vi "receiveUdp.vi"() -> ()   [LabVIEW 2021]
uses:
  Jump_Globals.vi
  senzorji.vi
  Jumps_Globals.vi
  Stevci_Globals.vi
  filePath.vi
  belezenje.vi
  <vilib>/express/express arith-compare/Formula/XNode/ExpressFormulaBlockNode.xnode
panel:
  out "Whole packet  3":string
  out "Whole packet  2":string
  out "Whole packet  1":string
  out "Whole packet 6  2":string
  out "Whole packet 5  2":string
  out "Whole packet  4":string
  out "Numeric":dbl
  out "appended path":path
  out "Jump ID 6":string
  out "Jump time  6":string
  out "Flight time 6":string
  out "Battery  6":string
  out "Sensor ID   6":string
  out "Packet Time 6":string
  out "appended path 6":path
  out "Jump ID 5":string
  out "Jump time  5":string
  out "Flight time 5":string
  out "Battery  5":string
  out "Sensor ID   5":string
  out "Packet Time 5":string
  out "appended path 5":path
  out "Jump ID 4":string
  out "Jump time  4":string
  out "Flight time 4":string
  out "Battery  4":string
  out "Sensor ID   4":string
  out "Packet Time 4":string
  out "appended path 4":path
  out "Jump ID 3":string
  out "Jump time  3":string
  out "Flight time 3":string
  out "Battery  3":string
  out "Sensor ID   3":string
  out "Packet Time 3":string
  out "Jump ID 2":string
  out "Jump time  2":string
  out "Flight time 2":string
  out "Battery  2":string
  out "Sensor ID   2":string
  out "Packet Time  2":string
  out "appended path 2":path
  out "Packet Time":string
  out "Sensor ID":string
  out "Whole packet":string
  out "Battery":string
  out "Flight time":string
  out "Jump time":string
  out "Jump ID":string
  in  "Stop":bool
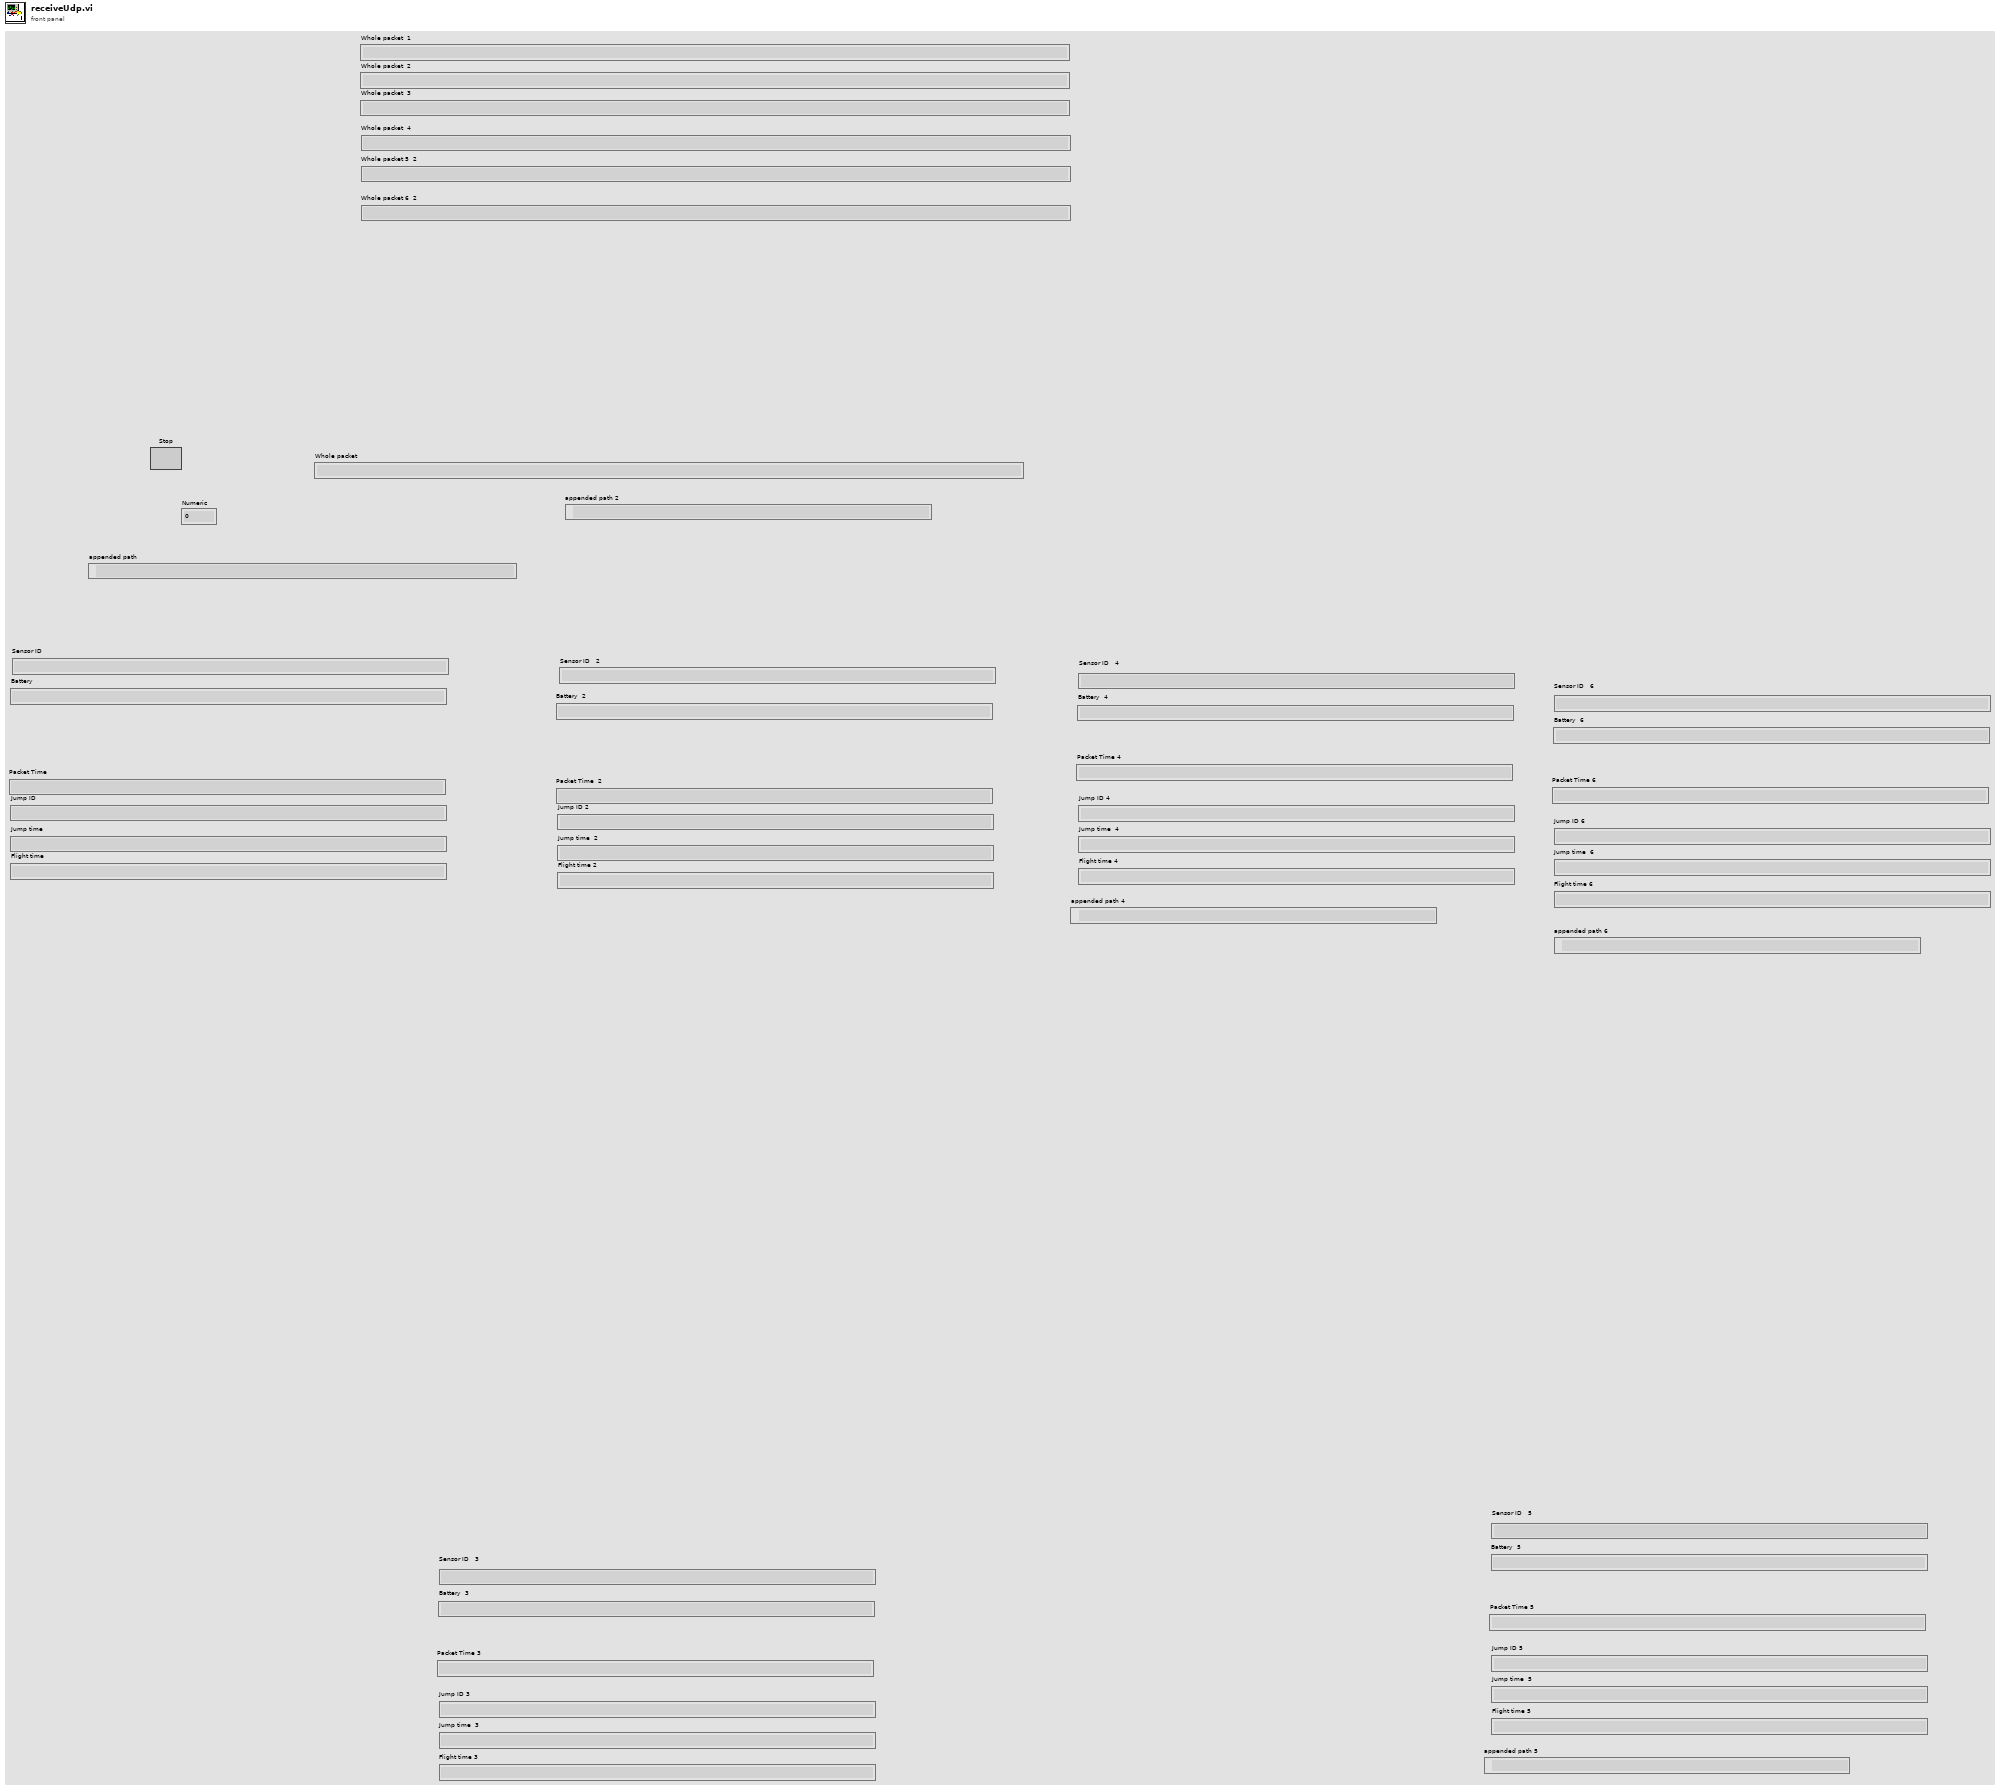
[diagram p1: front panel]
types:
  T1 = enum16{"open", "open or create", "create or replace", "create", "open (read-only)"}
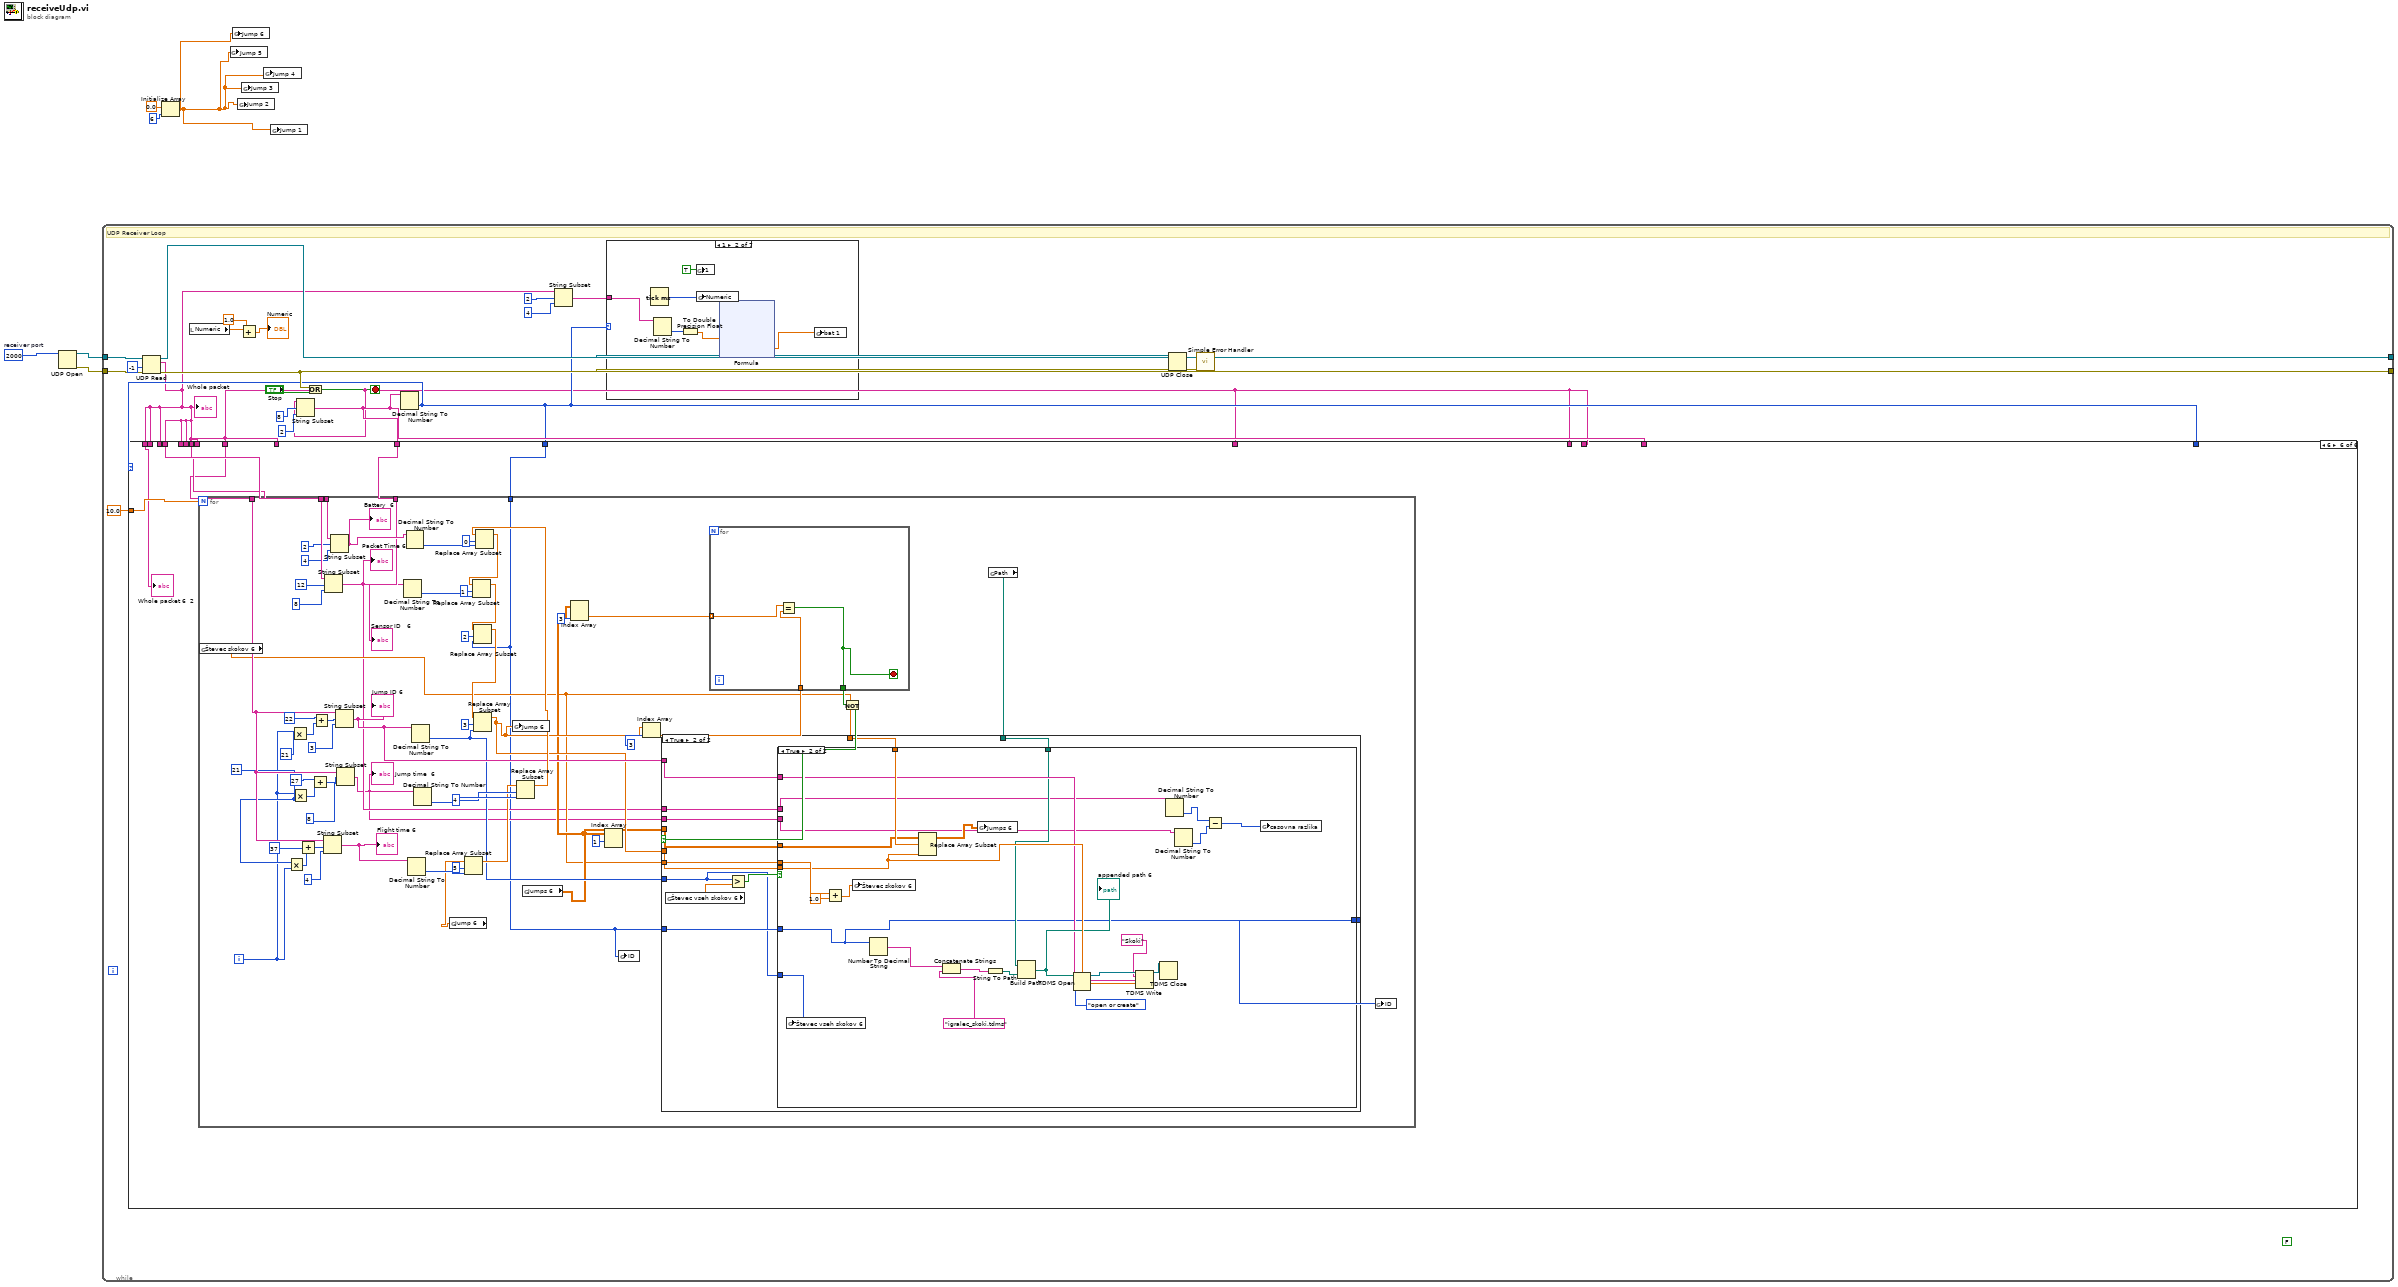
[diagram p0: block diagram]
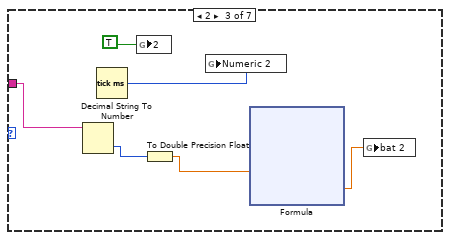
[diagram p3: hidden frame]
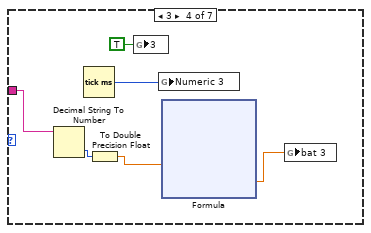
[diagram p4: hidden frame]
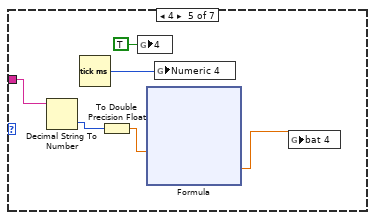
[diagram p5: hidden frame]
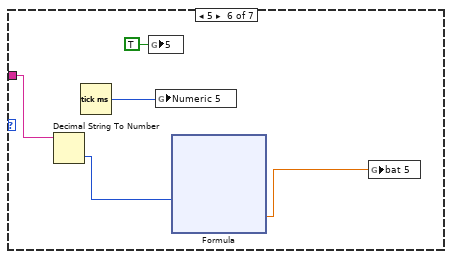
[diagram p6: hidden frame]
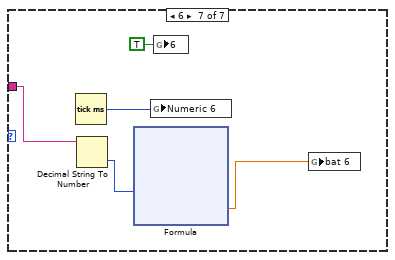
[diagram p7: hidden frame]
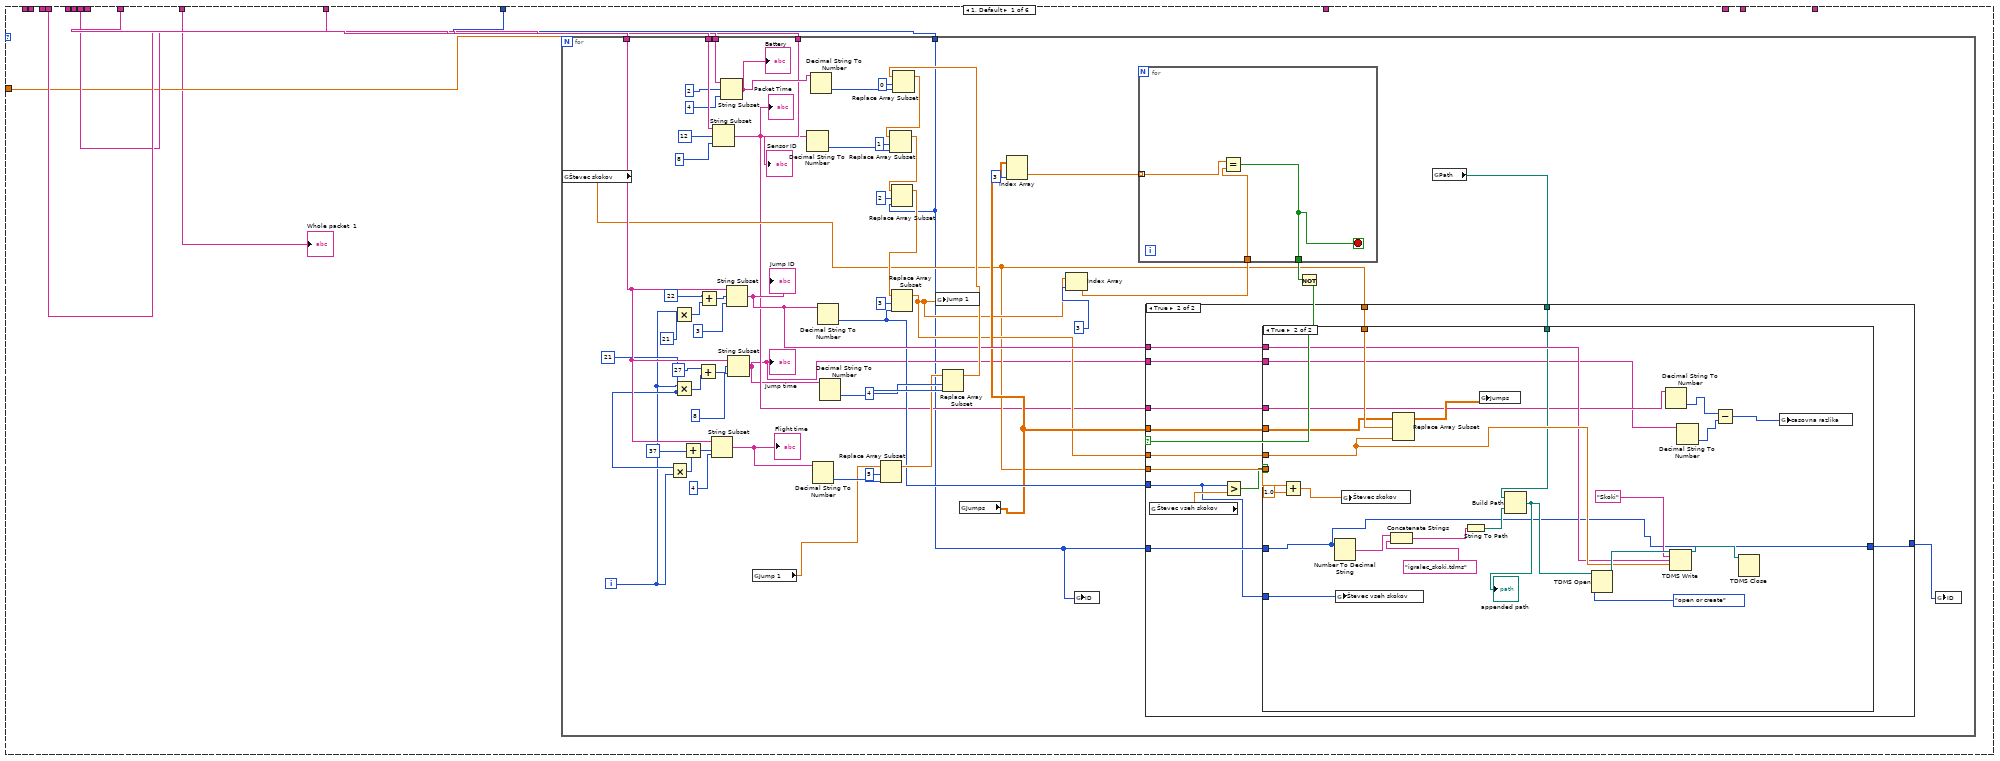
[diagram p8: hidden frame]
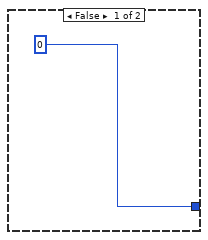
[diagram p9: hidden frame]
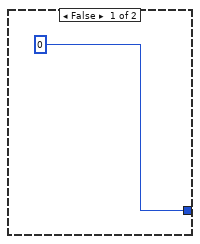
[diagram p10: hidden frame]
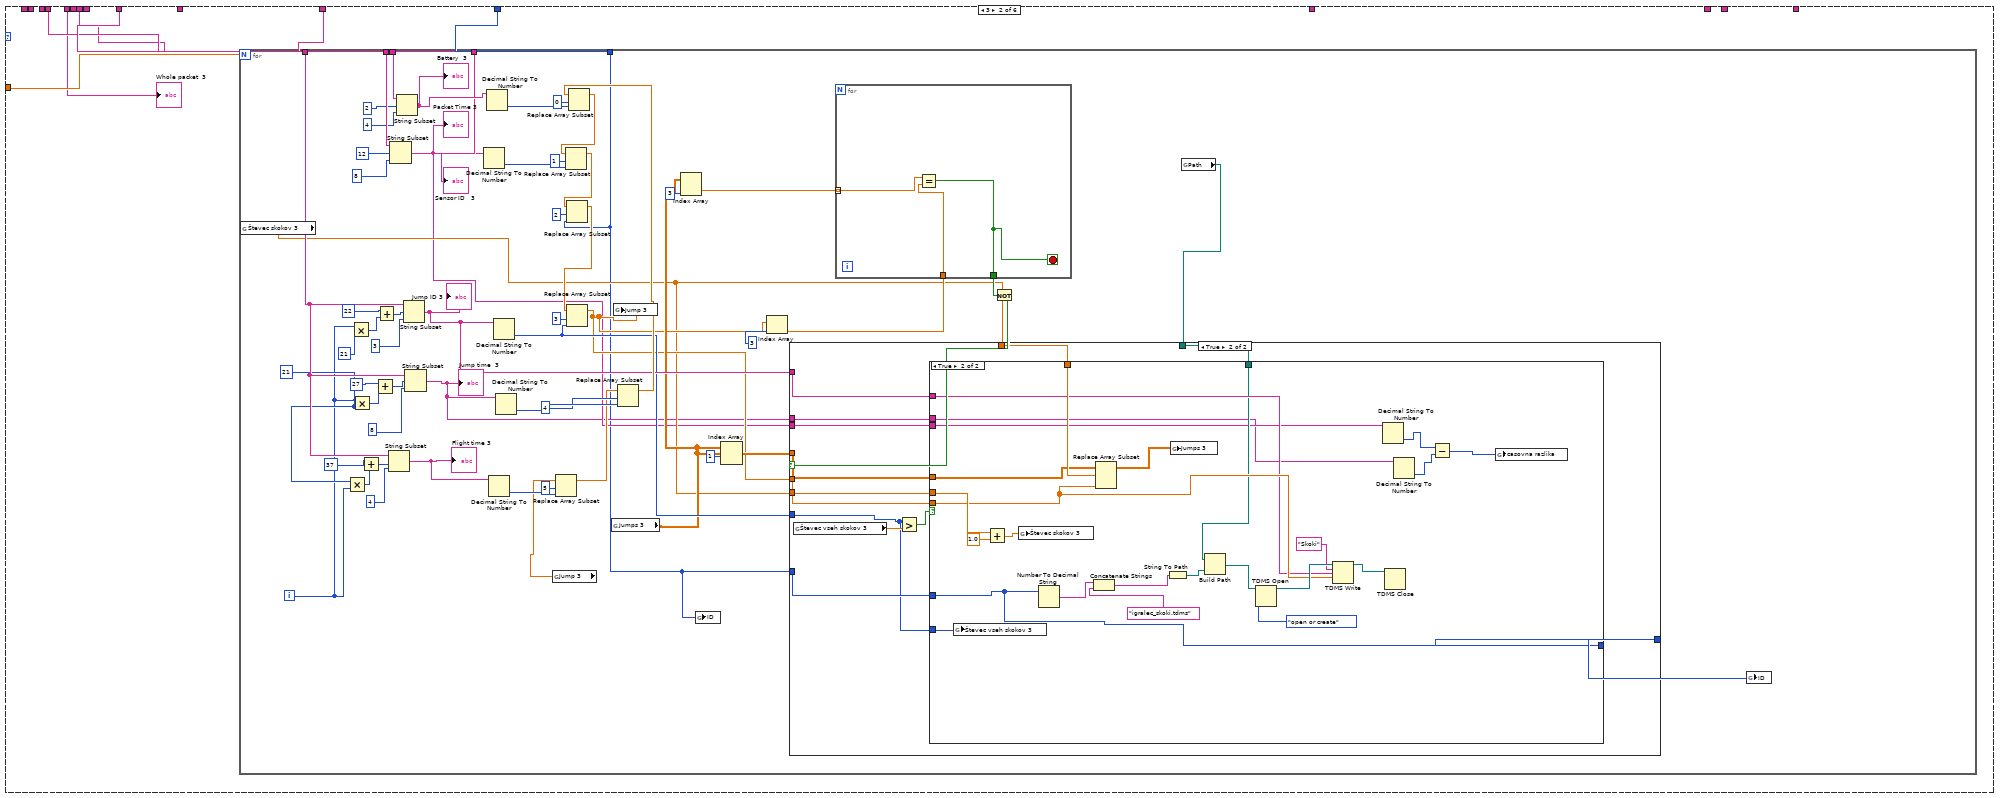
[diagram p11: hidden frame]
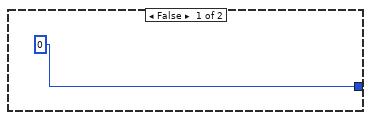
[diagram p12: hidden frame]
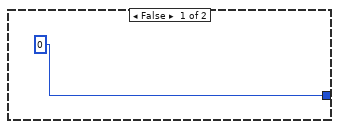
[diagram p13: hidden frame]
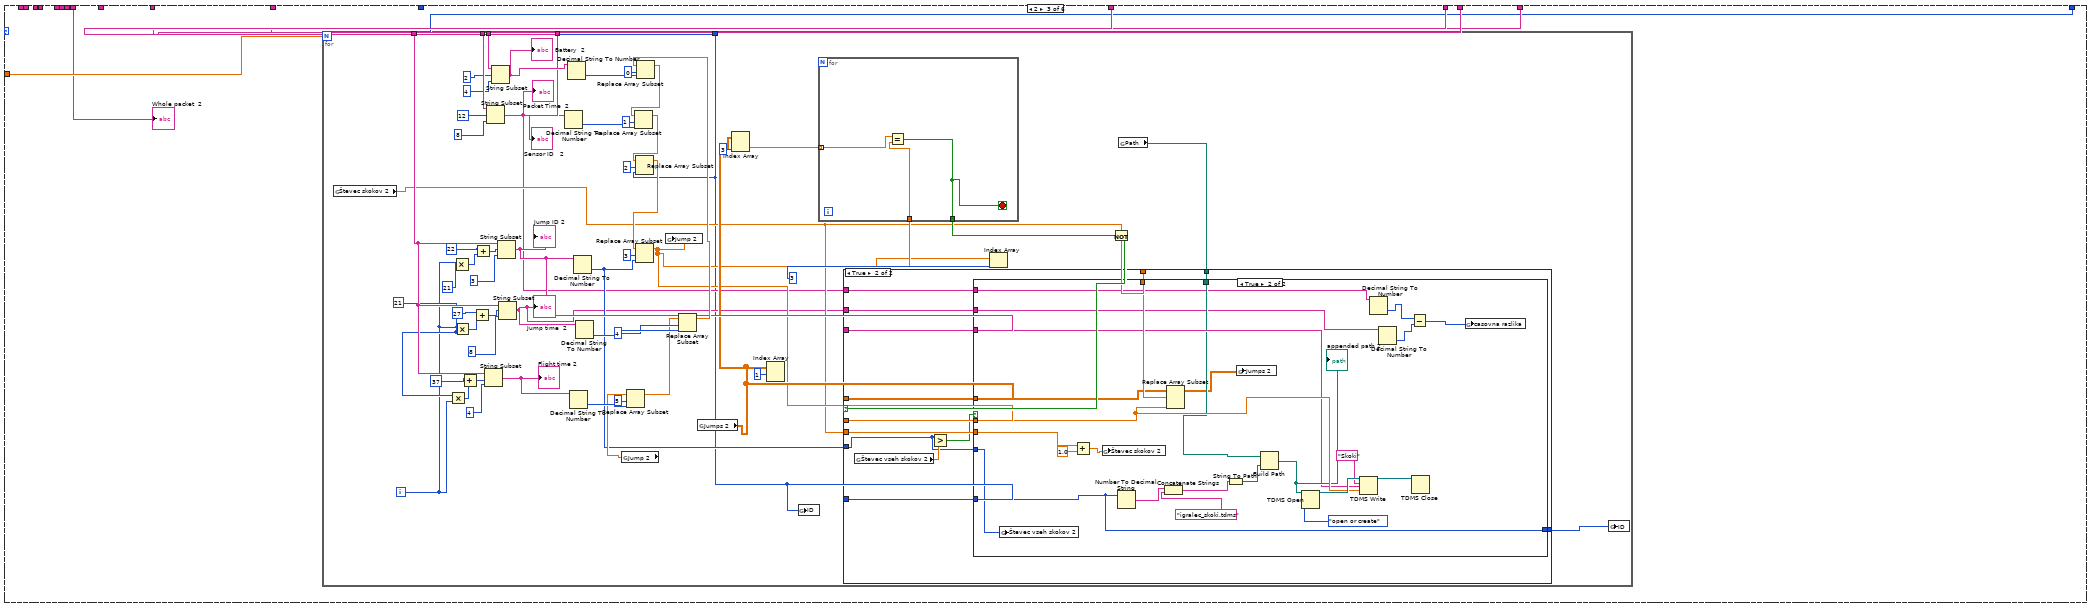
[diagram p14: hidden frame]
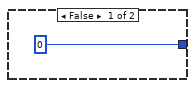
[diagram p15: hidden frame]
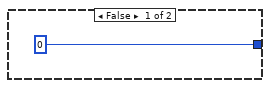
[diagram p16: hidden frame]
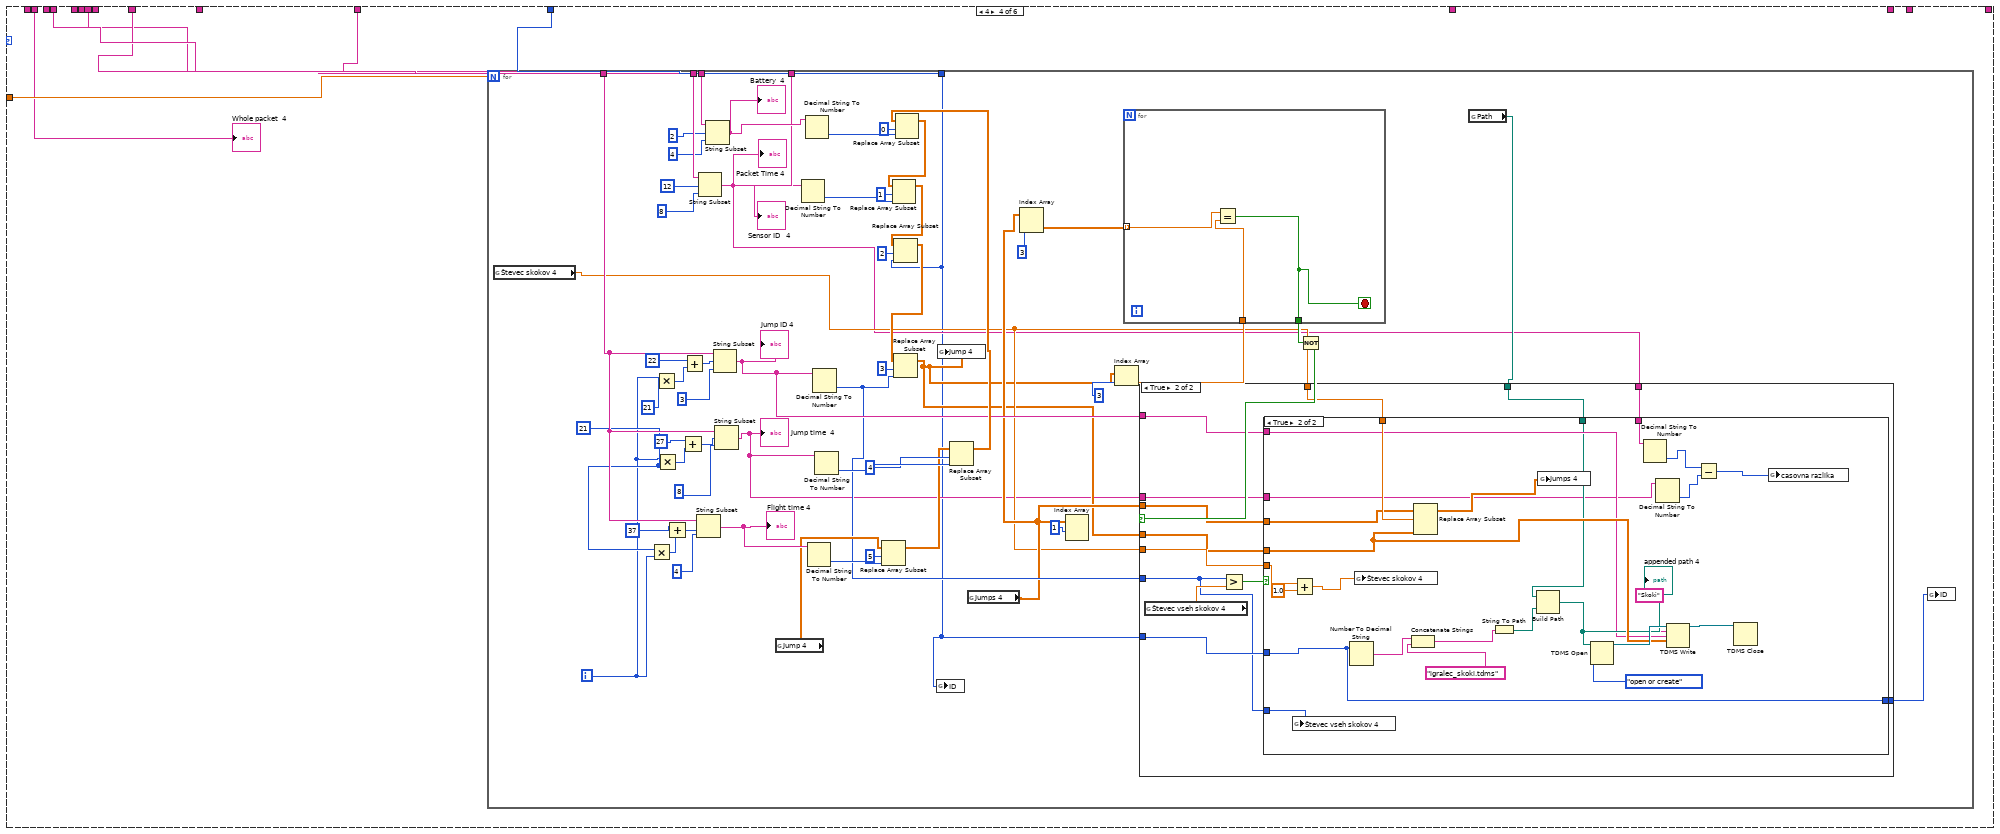
[diagram p17: hidden frame]
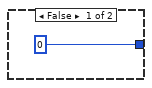
[diagram p18: hidden frame]
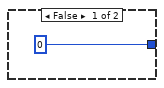
[diagram p19: hidden frame]
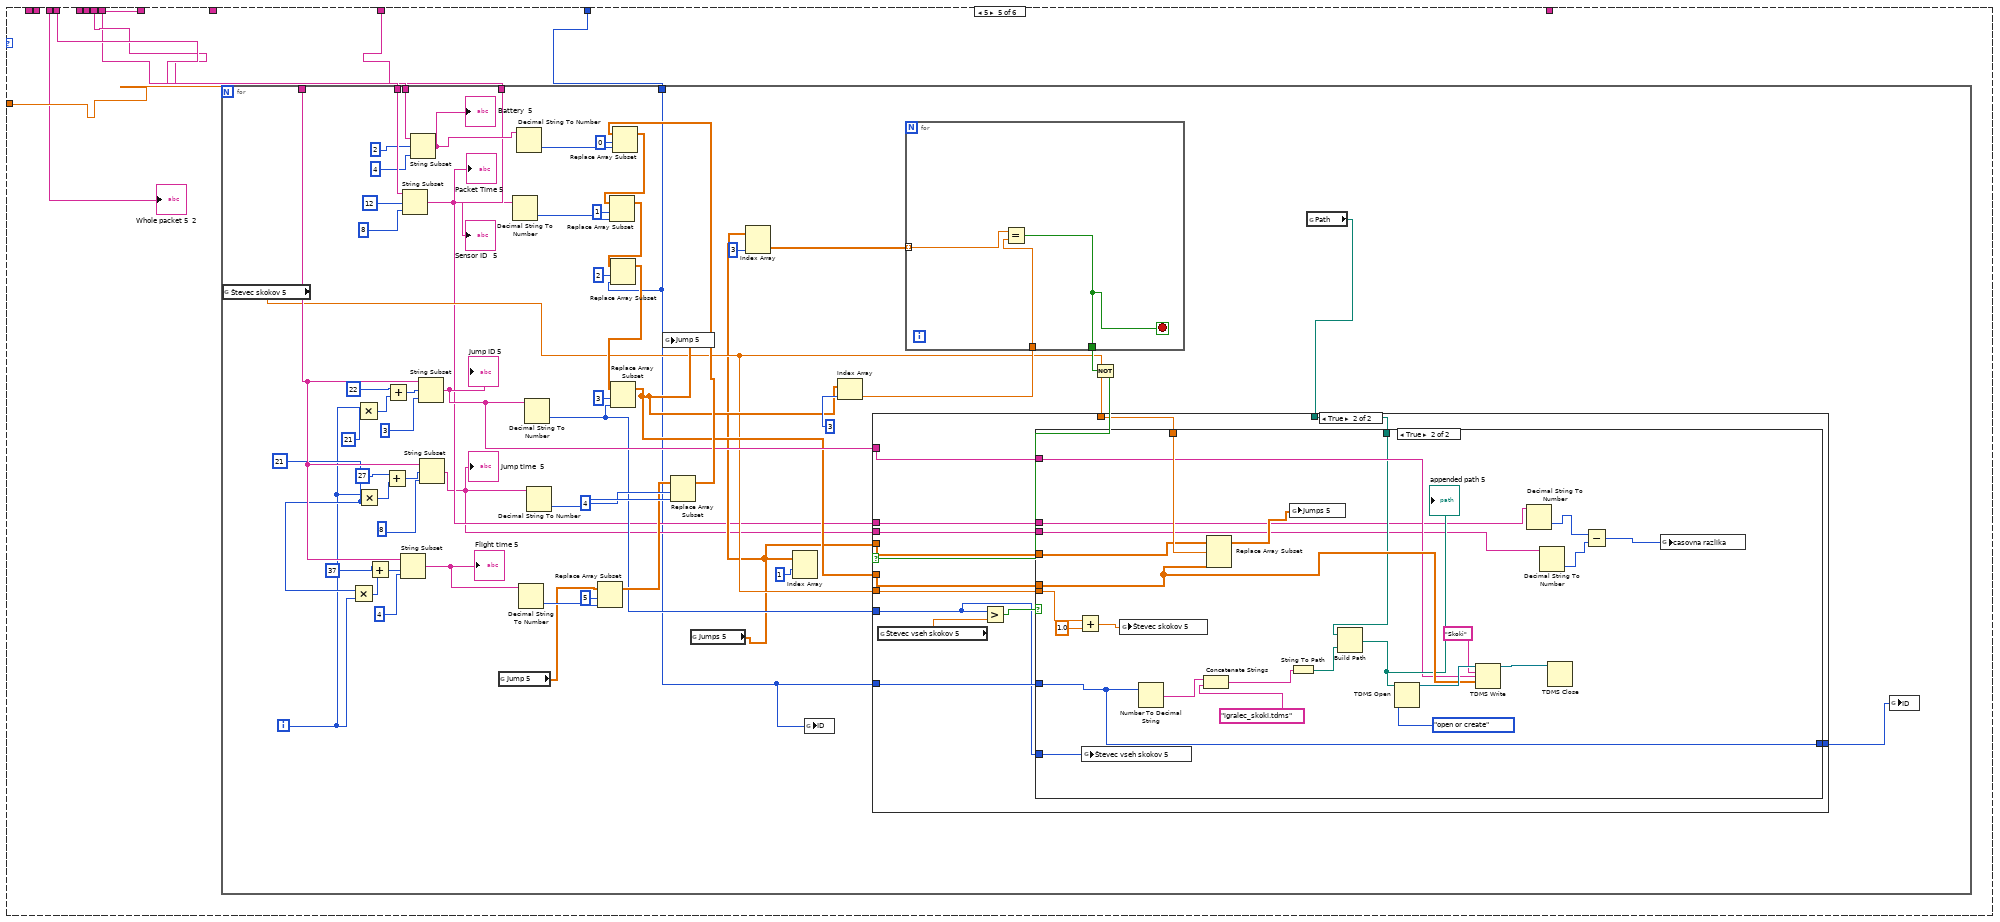
[diagram p20: hidden frame]
diagram:
  w2 = u16 2000  # receiver port
  n1 = UDP Open(11:w2) -> (port=w3:refnum<k16>, 0:w4:errorcluster)  [unwired: 4 in, 1 out]
  n2 = while {
    tunnel: w3 -> [w28]
    tunnel: [w24] -> w7
    tunnel: w4 -> [w25]
    tunnel: [w23] -> w5
    stop <- w26 stop-if-true
    (unwired) FALSE
    # "UDP Receiver Loop"
    n3 = UDP Read(connection ID=w28, timeout ms (25000)=-1, 8:w25) -> (data out=w10:string, error out=w23:errorcluster, 3:w24:refnum<k16>)  [unwired: 3 out]
    "Whole packet" <- w10
    n4 = local read "Numeric"() -> (w13:dbl)
    n5 = Add(x=w13, y=1.0) -> (x+y=→"Numeric":dbl)
    n6 = String Subset(string=w10, offset (0)=8, length (rest)=2) -> (substring=w20:string)
    n7 = Or(x=w23, y="Stop") -> (x .or. y?=w26:bool)
    n8 = Decimal String To Number(string=w20) -> (number=w17:i32)  [unwired: 2 in, 1 out]
    n9 = case shown="6" w17 {
      tunnel: w10 -> [w117 w223 _ w438 w546 w653]
      tunnel: w10 -> [w116 w222 _ w436 w548 w656]
      tunnel: w10 -> [w115 w221 _ w439 w547 w654]
      tunnel: w20 -> [w114 w220 _ w437 w544 w652]
      tunnel: w17 -> [w113 w224 _ w440 w545 w655]
      tunnel: w10 -> [_ _ w332 _ _ _]
      tunnel: w10 -> [_ _ w331 _ _ _]
      tunnel: w10 -> [_ _ w330 _ _ _]
      tunnel: w20 -> [_ _ w329 _ _ _]
      tunnel: w17 -> [_ _ w328 _ _ _]
      tunnel: 10.0 ("Numeric") -> [w112 w219 w327 w435 w543 w651]
      tunnel: w10 -> [w111 _ _ _ _ _]
      tunnel: w10 -> [_ _ _ _ _ _]
      tunnel: w10 -> [_ w218 _ _ _ _]
      tunnel: w10 -> [_ _ w326 _ _ _]
      tunnel: w10 -> [_ _ _ w434 _ _]
      tunnel: w10 -> [_ _ _ _ w542 _]
      tunnel: w10 -> [_ _ _ _ _ w650]
      frame 1, Default {
        n10 = for {
          N: w112 -> [_]
          tunnel: w117 -> [w171]
          tunnel: w116 -> [w148]
          tunnel: w115 -> [w145]
          tunnel: w114 -> [w128]
          tunnel: w113 -> [w118]
          i -> [w131]
          w163 = 21
          n11 = global read "Stevci_Globals.vi" "Števec skokov"() -> (w122:dbl)
          n12 = Multiply(x=w163, y=w131) -> (x*y=w166:i32)
          n13 = Multiply(x=21, y=w131) -> (x*y=w168:i32)
          n14 = Multiply(x=w131, y=w163) -> (x*y=w170:i32)
          n15 = Add(x=37, y=w166) -> (x+y=w165:i32)
          n16 = Add(x=27, y=w170) -> (x+y=w161:i32)
          n17 = Add(x=22, y=w168) -> (x+y=w160:i32)
          n18 = String Subset(string=w171, offset (0)=w165, length (rest)=4) -> (substring=w159:string)
          "Flight time" <- w159
          n19 = String Subset(string=w148, offset (0)=12, length (rest)=8) -> (substring=w120:string)
          "Packet Time" <- w120
          n20 = String Subset(string=w145, offset (0)=2, length (rest)=4) -> (substring=w137:string)
          "Battery" <- w137
          n21 = String Subset(string=w171, offset (0)=w160, length (rest)=3) -> (substring=w129:string)
          "Jump ID" <- w129
          n22 = String Subset(string=w171, offset (0)=w161, length (rest)=8) -> (substring=w119:string)
          "Jump time" <- w119
          n23 = global read "Jump_Globals.vi" "Jump 1"() -> (w124:dbl[])
          n24 = Decimal String To Number(string=w120) -> (number=w152:i32)  [unwired: 2 in, 1 out]
          n25 = Decimal String To Number(string=w137) -> (number=w151:i32)  [unwired: 2 in, 1 out]
          n26 = Decimal String To Number(string=w159) -> (number=w157:i32)  [unwired: 2 in, 1 out]
          n27 = Decimal String To Number(string=w129) -> (number=w127:i32)  [unwired: 2 in, 1 out]
          n28 = Decimal String To Number(string=w119) -> (number=w158:i32)  [unwired: 2 in, 1 out]
          n29 = Replace Array Subset(array=w124, new element=w157, index=5) -> (w153:dbl[])
          n30 = Replace Array Subset(array=w153, new element=w158, index=4) -> (w144:dbl[])
          n31 = Replace Array Subset(array=w144, new element=w151, index=0) -> (w143:dbl[])
          n32 = Replace Array Subset(array=w143, new element=w152, index=1) -> (w142:dbl[])
          n33 = Replace Array Subset(array=w142, new element=w118, index=2) -> (w141:dbl[])
          n34 = Replace Array Subset(array=w141, new element=w127, index=3) -> (w123:dbl[])
          n35 = global write "Jump_Globals.vi" "Jump 1"(w123) -> ()
          n36 = global read "Jumps_Globals.vi" "Jumps"() -> (w125:dbl[][])
          n37 = Index Array(array=w125, index (col)=3 ("disabled index (col)")) -> (element=w135:dbl[])  [unwired: 1 in]
          n38 = Index Array(array=w123, index=3) -> (element=w133:dbl)
          n39 = global write "belezenje.vi" "ID"(w118) -> ()
          n40 = for {
            tunnel: w135 -> [w217] mode=indexing
            tunnel: w133 -> [w216]
            tunnel: [w215] -> w132
            stop <- w215 stop-if-true
            n41 = Equal?(x=w217, y=w216) -> (x = y?=w215:bool)
          }
          n42 = Not(x=w132) -> (.not. x?=w130:bool)
          n43 = global read "filePath.vi" "Path"() -> (w121:path)
          n44 = case shown="True" w130 {
            tunnel: w125 -> [_ w186]
            tunnel: w123 -> [_ w185]
            tunnel: w122 -> [_ w188]
            tunnel: w122 -> [_ w187]
            tunnel: w129 -> [_ w184]
            tunnel: w118 -> [_ w183]
            tunnel: w121 -> [_ w182]
            tunnel: w127 -> [_ w179]
            tunnel: [0 w178] -> w126
            tunnel: w120 -> [_ w177]
            tunnel: w119 -> [_ w176]
            frame False {
            }
            frame True {
              n45 = global read "Stevci_Globals.vi" "Števec vseh skokov"() -> (w181:dbl)
              n46 = Greater?(x=w179, y=w181) -> (0:w180:bool)
              n47 = case shown="True" w180 {
                tunnel: w188 -> [_ w214]
                tunnel: w187 -> [_ w213]
                tunnel: w186 -> [_ w208]
                tunnel: w185 -> [_ w207]
                tunnel: w184 -> [_ w204]
                tunnel: w183 -> [_ w195]
                tunnel: w182 -> [_ w199]
                tunnel: w179 -> [_ w196]
                tunnel: [0 w195] -> w178
                tunnel: w177 -> [_ w191]
                tunnel: w176 -> [_ w190]
                frame False {
                }
                frame True {
                  n48 = Add(x=w213, y=1.0) -> (x+y=w197:dbl)
                  n49 = Number To Decimal String(number=w195) -> (decimal integer string=w203:string)  [unwired: 1 in]
                  n50 = global write "Stevci_Globals.vi" "Števec vseh skokov"(w196) -> ()
                  n51 = global write "Stevci_Globals.vi" "Števec skokov"(w197) -> ()
                  n52 = Concatenate Strings(w203, "igralec_skoki.tdms") -> (w201:string)
                  n53 = Replace Array Subset(array=w208, new element=w207, index (row)=w214) -> (w198:dbl[][])  [unwired: 1 in]
                  n54 = String To Path(string=w201) -> (path=w200:path)
                  n55 = global write "Jumps_Globals.vi" "Jumps"(w198) -> ()
                  n56 = Build Path(base path=w199, name or relative path=w200) -> (appended path=w206:path)
                  "appended path" <- w206
                  n57 = TDMS Open(10:T1."open or create" ("operation (0:open)"), 11:w206) -> (3:w211:refnum<k34>)  [unwired: 5 in, 1 out]
                  n58 = Decimal String To Number(string=w191) -> (number=w193:i32)  [unwired: 2 in, 1 out]
                  n59 = TDMS Write(0:w211, 5:"Skoki" ("group name in (Untitled)"), 7:w204, 9:w207) -> (4:w210:refnum<k34>)  [unwired: 2 in, 3 out]
                  n60 = Decimal String To Number(string=w190) -> (number=w192:i32)  [unwired: 2 in, 1 out]
                  n61 = Subtract(x=w193, y=w192) -> (x-y=w194:i32)
                  n62 = TDMS Close(11:w210) -> ()  [unwired: 1 in, 2 out]
                  n63 = global write "Stevci_Globals.vi" "casovna razlika"(w194) -> ()
                }
              }
            }
          }
          n64 = global write "belezenje.vi" "ID"(w126) -> ()
          "Sensor ID" <- w128
        }
        "Whole packet  1" <- w111
      }
      frame 3 {
        n65 = for {
          N: w219 -> [_]
          tunnel: w223 -> [w279]
          tunnel: w222 -> [w255]
          tunnel: w221 -> [w252]
          tunnel: w220 -> [w235]
          tunnel: w224 -> [w225]
          i -> [w238]
          w271 = 21
          n66 = global read "Stevci_Globals.vi" "Števec skokov 3"() -> (w229:dbl)
          n67 = Multiply(x=w271, y=w238) -> (x*y=w274:i32)
          n68 = Multiply(x=21, y=w238) -> (x*y=w276:i32)
          n69 = Multiply(x=w238, y=w271) -> (x*y=w278:i32)
          n70 = Add(x=37, y=w274) -> (x+y=w273:i32)
          n71 = Add(x=27, y=w278) -> (x+y=w269:i32)
          n72 = Add(x=22, y=w276) -> (x+y=w268:i32)
          n73 = String Subset(string=w279, offset (0)=w273, length (rest)=4) -> (substring=w267:string)
          "Flight time 3" <- w267
          n74 = String Subset(string=w255, offset (0)=12, length (rest)=8) -> (substring=w227:string)
          "Packet Time 3" <- w227
          n75 = String Subset(string=w252, offset (0)=2, length (rest)=4) -> (substring=w244:string)
          "Battery  3" <- w244
          n76 = String Subset(string=w279, offset (0)=w268, length (rest)=3) -> (substring=w236:string)
          "Jump ID 3" <- w236
          n77 = String Subset(string=w279, offset (0)=w269, length (rest)=8) -> (substring=w226:string)
          "Jump time  3" <- w226
          n78 = Decimal String To Number(string=w227) -> (number=w259:i32)  [unwired: 2 in, 1 out]
          n79 = Decimal String To Number(string=w244) -> (number=w258:i32)  [unwired: 2 in, 1 out]
          n80 = Decimal String To Number(string=w267) -> (number=w265:i32)  [unwired: 2 in, 1 out]
          n81 = Decimal String To Number(string=w236) -> (number=w233:i32)  [unwired: 2 in, 1 out]
          n82 = Decimal String To Number(string=w226) -> (number=w266:i32)  [unwired: 2 in, 1 out]
          n83 = global read "Jump_Globals.vi" "Jump 3"() -> (w234:dbl[])
          n84 = Replace Array Subset(array=w234, new element=w265, index=5) -> (w261:dbl[])
          n85 = global read "Jumps_Globals.vi" "Jumps 3"() -> (w231:dbl[][])
          n86 = Replace Array Subset(array=w261, new element=w266, index=4) -> (w251:dbl[])
          n87 = Replace Array Subset(array=w251, new element=w258, index=0) -> (w250:dbl[])
          n88 = Replace Array Subset(array=w250, new element=w259, index=1) -> (w249:dbl[])
          n89 = Replace Array Subset(array=w249, new element=w225, index=2) -> (w248:dbl[])
          n90 = Replace Array Subset(array=w248, new element=w233, index=3) -> (w230:dbl[])
          n91 = global write "Jump_Globals.vi" "Jump 3"(w230) -> ()
          n92 = Index Array(array=w231, index (col)=3 ("disabled index (col)")) -> (element=w242:dbl[])  [unwired: 1 in]
          n93 = global write "belezenje.vi" "ID"(w225) -> ()
          n94 = Index Array(array=w231, index (row)=1) -> ()  [unwired: 1 in, 1 out]
          n95 = Index Array(array=w230, index=3) -> (element=w240:dbl)
          n96 = for {
            tunnel: w242 -> [w325] mode=indexing
            tunnel: w240 -> [w324]
            tunnel: [w323] -> w239
            stop <- w323 stop-if-true
            n97 = Equal?(x=w325, y=w324) -> (x = y?=w323:bool)
          }
          n98 = Not(x=w239) -> (.not. x?=w237:bool)
          n99 = global read "filePath.vi" "Path"() -> (w228:path)
          n100 = case shown="True" w237 {
            tunnel: w231 -> [_ w294]
            tunnel: w230 -> [_ w293]
            tunnel: w229 -> [_ w296]
            tunnel: w229 -> [_ w295]
            tunnel: w236 -> [_ w292]
            tunnel: w225 -> [_ w291]
            tunnel: w228 -> [_ w290]
            tunnel: w233 -> [_ w287]
            tunnel: [0 w286] -> w232
            tunnel: w227 -> [_ w285]
            tunnel: w226 -> [_ w284]
            frame False {
            }
            frame True {
              n101 = global read "Stevci_Globals.vi" "Števec vseh skokov 3"() -> (w289:dbl)
              n102 = Greater?(x=w287, y=w289) -> (0:w288:bool)
              n103 = case shown="True" w288 {
                tunnel: w296 -> [_ w322]
                tunnel: w295 -> [_ w321]
                tunnel: w294 -> [_ w316]
                tunnel: w293 -> [_ w315]
                tunnel: w292 -> [_ w312]
                tunnel: w291 -> [_ w303]
                tunnel: w290 -> [_ w307]
                tunnel: w287 -> [_ w305]
                tunnel: [0 w303] -> w286
                tunnel: w285 -> [_ w299]
                tunnel: w284 -> [_ w298]
                frame False {
                }
                frame True {
                  n104 = global write "Stevci_Globals.vi" "Števec vseh skokov 3"(w305) -> ()
                  n105 = Add(x=w321, y=1.0) -> (x+y=w304:dbl)
                  n106 = global write "Stevci_Globals.vi" "Števec skokov 3"(w304) -> ()
                  n107 = Number To Decimal String(number=w303) -> (decimal integer string=w311:string)  [unwired: 1 in]
                  n108 = Concatenate Strings(w311, "igralec_skoki.tdms") -> (w309:string)
                  n109 = Replace Array Subset(array=w316, new element=w315, index (row)=w322) -> (w306:dbl[][])  [unwired: 1 in]
                  n110 = String To Path(string=w309) -> (path=w308:path)
                  n111 = global write "Jumps_Globals.vi" "Jumps 3"(w306) -> ()
                  n112 = Build Path(base path=w307, name or relative path=w308) -> (appended path=w314:path)
                  n113 = TDMS Open(10:T1."open or create" ("operation (0:open)"), 11:w314) -> (3:w319:refnum<k34>)  [unwired: 5 in, 1 out]
                  n114 = TDMS Write(0:w319, 5:"Skoki" ("group name in (Untitled)"), 7:w312, 9:w315) -> (4:w318:refnum<k34>)  [unwired: 2 in, 3 out]
                  n115 = Decimal String To Number(string=w299) -> (number=w301:i32)  [unwired: 2 in, 1 out]
                  n116 = TDMS Close(11:w318) -> ()  [unwired: 1 in, 2 out]
                  n117 = Decimal String To Number(string=w298) -> (number=w300:i32)  [unwired: 2 in, 1 out]
                  n118 = Subtract(x=w301, y=w300) -> (x-y=w302:i32)
                  n119 = global write "Stevci_Globals.vi" "casovna razlika"(w302) -> ()
                }
              }
            }
          }
          n120 = global write "belezenje.vi" "ID"(w232) -> ()
          "Sensor ID   3" <- w235
        }
        "Whole packet  3" <- w218
      }
      frame 2 {
        n121 = for {
          N: w327 -> [_]
          tunnel: w332 -> [w387]
          tunnel: w331 -> [w363]
          tunnel: w330 -> [w360]
          tunnel: w329 -> [w343]
          tunnel: w328 -> [w333]
          i -> [w346]
          w379 = 21
          n122 = global read "Stevci_Globals.vi" "Števec skokov 2"() -> (w337:dbl)
          n123 = Multiply(x=w379, y=w346) -> (x*y=w382:i32)
          n124 = Multiply(x=21, y=w346) -> (x*y=w384:i32)
          n125 = Multiply(x=w346, y=w379) -> (x*y=w386:i32)
          n126 = Add(x=37, y=w382) -> (x+y=w381:i32)
          n127 = Add(x=27, y=w386) -> (x+y=w377:i32)
          n128 = Add(x=22, y=w384) -> (x+y=w376:i32)
          n129 = String Subset(string=w387, offset (0)=w381, length (rest)=4) -> (substring=w375:string)
          "Flight time 2" <- w375
          n130 = String Subset(string=w363, offset (0)=12, length (rest)=8) -> (substring=w335:string)
          "Packet Time  2" <- w335
          n131 = String Subset(string=w360, offset (0)=2, length (rest)=4) -> (substring=w352:string)
          "Battery  2" <- w352
          n132 = String Subset(string=w387, offset (0)=w376, length (rest)=3) -> (substring=w344:string)
          "Jump ID 2" <- w344
          n133 = String Subset(string=w387, offset (0)=w377, length (rest)=8) -> (substring=w334:string)
          "Jump time  2" <- w334
          n134 = Decimal String To Number(string=w335) -> (number=w367:i32)  [unwired: 2 in, 1 out]
          n135 = Decimal String To Number(string=w352) -> (number=w366:i32)  [unwired: 2 in, 1 out]
          n136 = Decimal String To Number(string=w375) -> (number=w373:i32)  [unwired: 2 in, 1 out]
          n137 = Decimal String To Number(string=w344) -> (number=w341:i32)  [unwired: 2 in, 1 out]
          n138 = Decimal String To Number(string=w334) -> (number=w374:i32)  [unwired: 2 in, 1 out]
          n139 = global read "Jump_Globals.vi" "Jump 2"() -> (w342:dbl[])
          n140 = Replace Array Subset(array=w342, new element=w373, index=5) -> (w369:dbl[])
          n141 = Replace Array Subset(array=w369, new element=w374, index=4) -> (w359:dbl[])
          n142 = Replace Array Subset(array=w359, new element=w366, index=0) -> (w358:dbl[])
          n143 = Replace Array Subset(array=w358, new element=w367, index=1) -> (w357:dbl[])
          n144 = Replace Array Subset(array=w357, new element=w333, index=2) -> (w356:dbl[])
          n145 = Replace Array Subset(array=w356, new element=w341, index=3) -> (w338:dbl[])
          n146 = global write "Jump_Globals.vi" "Jump 2"(w338) -> ()
          n147 = global read "Jumps_Globals.vi" "Jumps 2"() -> (w339:dbl[][])
          n148 = Index Array(array=w339, index (col)=3 ("disabled index (col)")) -> (element=w350:dbl[])  [unwired: 1 in]
          n149 = Index Array(array=w339, index (row)=1) -> ()  [unwired: 1 in, 1 out]
          n150 = global write "belezenje.vi" "ID"(w333) -> ()
          n151 = Index Array(array=w338, index=3) -> (element=w348:dbl)
          n152 = for {
            tunnel: w350 -> [w433] mode=indexing
            tunnel: w348 -> [w432]
            tunnel: [w431] -> w347
            stop <- w431 stop-if-true
            n153 = Equal?(x=w433, y=w432) -> (x = y?=w431:bool)
          }
          n154 = Not(x=w347) -> (.not. x?=w345:bool)
          n155 = global read "filePath.vi" "Path"() -> (w336:path)
          n156 = case shown="True" w345 {
            tunnel: w339 -> [_ w402]
            tunnel: w338 -> [_ w401]
            tunnel: w337 -> [_ w404]
            tunnel: w337 -> [_ w403]
            tunnel: w344 -> [_ w400]
            tunnel: w333 -> [_ w399]
            tunnel: w336 -> [_ w398]
            tunnel: w341 -> [_ w395]
            tunnel: [0 w394] -> w340
            tunnel: w335 -> [_ w393]
            tunnel: w334 -> [_ w392]
            frame False {
            }
            frame True {
              n157 = global read "Stevci_Globals.vi" "Števec vseh skokov 2"() -> (w397:dbl)
              n158 = Greater?(x=w395, y=w397) -> (0:w396:bool)
              n159 = case shown="True" w396 {
                tunnel: w404 -> [_ w430]
                tunnel: w403 -> [_ w429]
                tunnel: w402 -> [_ w424]
                tunnel: w401 -> [_ w423]
                tunnel: w400 -> [_ w420]
                tunnel: w399 -> [_ w411]
                tunnel: w398 -> [_ w415]
                tunnel: w395 -> [_ w413]
                tunnel: [0 w411] -> w394
                tunnel: w393 -> [_ w407]
                tunnel: w392 -> [_ w406]
                frame False {
                }
                frame True {
                  n160 = global write "Stevci_Globals.vi" "Števec vseh skokov 2"(w413) -> ()
                  n161 = Add(x=w429, y=1.0) -> (x+y=w412:dbl)
                  n162 = global write "Stevci_Globals.vi" "Števec skokov 2"(w412) -> ()
                  n163 = Number To Decimal String(number=w411) -> (decimal integer string=w419:string)  [unwired: 1 in]
                  n164 = Concatenate Strings(w419, "igralec_skoki.tdms") -> (w417:string)
                  n165 = Replace Array Subset(array=w424, new element=w423, index (row)=w430) -> (w414:dbl[][])  [unwired: 1 in]
                  n166 = String To Path(string=w417) -> (path=w416:path)
                  n167 = global write "Jumps_Globals.vi" "Jumps 2"(w414) -> ()
                  n168 = Build Path(base path=w415, name or relative path=w416) -> (appended path=w422:path)
                  "appended path 2" <- w422
                  n169 = TDMS Open(10:T1."open or create" ("operation (0:open)"), 11:w422) -> (3:w427:refnum<k34>)  [unwired: 5 in, 1 out]
                  n170 = TDMS Write(0:w427, 5:"Skoki" ("group name in (Untitled)"), 7:w420, 9:w423) -> (4:w426:refnum<k34>)  [unwired: 2 in, 3 out]
                  n171 = Decimal String To Number(string=w407) -> (number=w409:i32)  [unwired: 2 in, 1 out]
                  n172 = Decimal String To Number(string=w406) -> (number=w408:i32)  [unwired: 2 in, 1 out]
                  n173 = Subtract(x=w409, y=w408) -> (x-y=w410:i32)
                  n174 = TDMS Close(11:w426) -> ()  [unwired: 1 in, 2 out]
                  n175 = global write "Stevci_Globals.vi" "casovna razlika"(w410) -> ()
                }
              }
            }
          }
          n176 = global write "belezenje.vi" "ID"(w340) -> ()
          "Sensor ID   2" <- w343
        }
        "Whole packet  2" <- w326
      }
      frame 4 {
        n177 = for {
          N: w435 -> [_]
          tunnel: w438 -> [w495]
          tunnel: w436 -> [w471]
          tunnel: w439 -> [w468]
          tunnel: w437 -> [w451]
          tunnel: w440 -> [w441]
          i -> [w454]
          w487 = 21
          n178 = global read "Stevci_Globals.vi" "Števec skokov 4"() -> (w446:dbl)
          n179 = Multiply(x=w487, y=w454) -> (x*y=w490:i32)
          n180 = Multiply(x=21, y=w454) -> (x*y=w492:i32)
          n181 = Multiply(x=w454, y=w487) -> (x*y=w494:i32)
          n182 = Add(x=37, y=w490) -> (x+y=w489:i32)
          n183 = Add(x=27, y=w494) -> (x+y=w485:i32)
          n184 = Add(x=22, y=w492) -> (x+y=w484:i32)
          n185 = String Subset(string=w495, offset (0)=w489, length (rest)=4) -> (substring=w483:string)
          "Flight time 4" <- w483
          n186 = String Subset(string=w471, offset (0)=12, length (rest)=8) -> (substring=w443:string)
          "Packet Time 4" <- w443
          n187 = String Subset(string=w468, offset (0)=2, length (rest)=4) -> (substring=w460:string)
          "Battery  4" <- w460
          n188 = String Subset(string=w495, offset (0)=w484, length (rest)=3) -> (substring=w452:string)
          "Jump ID 4" <- w452
          n189 = String Subset(string=w495, offset (0)=w485, length (rest)=8) -> (substring=w442:string)
          "Jump time  4" <- w442
          n190 = global read "Jump_Globals.vi" "Jump 4"() -> (w450:dbl[])
          n191 = Decimal String To Number(string=w443) -> (number=w475:i32)  [unwired: 2 in, 1 out]
          n192 = Decimal String To Number(string=w460) -> (number=w474:i32)  [unwired: 2 in, 1 out]
          n193 = Decimal String To Number(string=w483) -> (number=w481:i32)  [unwired: 2 in, 1 out]
          n194 = Decimal String To Number(string=w452) -> (number=w449:i32)  [unwired: 2 in, 1 out]
          n195 = Decimal String To Number(string=w442) -> (number=w482:i32)  [unwired: 2 in, 1 out]
          n196 = Replace Array Subset(array=w450, new element=w481, index=5) -> (w477:dbl[])
          n197 = global write "belezenje.vi" "ID"(w441) -> ()
          n198 = Replace Array Subset(array=w477, new element=w482, index=4) -> (w467:dbl[])
          n199 = Replace Array Subset(array=w467, new element=w474, index=0) -> (w466:dbl[])
          n200 = Replace Array Subset(array=w466, new element=w475, index=1) -> (w465:dbl[])
          n201 = Replace Array Subset(array=w465, new element=w441, index=2) -> (w464:dbl[])
          n202 = Replace Array Subset(array=w464, new element=w449, index=3) -> (w445:dbl[])
          n203 = global write "Jump_Globals.vi" "Jump 4"(w445) -> ()
          n204 = global read "Jumps_Globals.vi" "Jumps 4"() -> (w447:dbl[][])
          n205 = Index Array(array=w447, index (col)=3 ("disabled index (col)")) -> (element=w458:dbl[])  [unwired: 1 in]
          n206 = Index Array(array=w447, index (row)=1) -> ()  [unwired: 1 in, 1 out]
          n207 = Index Array(array=w445, index=3) -> (element=w456:dbl)
          n208 = for {
            tunnel: w458 -> [w541] mode=indexing
            tunnel: w456 -> [w540]
            tunnel: [w539] -> w455
            stop <- w539 stop-if-true
            n209 = Equal?(x=w541, y=w540) -> (x = y?=w539:bool)
          }
          n210 = Not(x=w455) -> (.not. x?=w453:bool)
          n211 = global read "filePath.vi" "Path"() -> (w444:path)
          n212 = case shown="True" w453 {
            tunnel: w447 -> [_ w510]
            tunnel: w445 -> [_ w509]
            tunnel: w446 -> [_ w512]
            tunnel: w446 -> [_ w511]
            tunnel: w452 -> [_ w508]
            tunnel: w441 -> [_ w507]
            tunnel: w444 -> [_ w506]
            tunnel: w449 -> [_ w503]
            tunnel: [0 w502] -> w448
            tunnel: w443 -> [_ w501]
            tunnel: w442 -> [_ w500]
            frame False {
            }
            frame True {
              n213 = global read "Stevci_Globals.vi" "Števec vseh skokov 4"() -> (w504:dbl)
              n214 = Greater?(x=w503, y=w504) -> (0:w505:bool)
              n215 = case shown="True" w505 {
                tunnel: w512 -> [_ w538]
                tunnel: w511 -> [_ w537]
                tunnel: w510 -> [_ w532]
                tunnel: w509 -> [_ w531]
                tunnel: w508 -> [_ w528]
                tunnel: w507 -> [_ w519]
                tunnel: w506 -> [_ w523]
                tunnel: w503 -> [_ w521]
                tunnel: [0 w519] -> w502
                tunnel: w501 -> [_ w515]
                tunnel: w500 -> [_ w514]
                frame False {
                }
                frame True {
                  n216 = global write "Stevci_Globals.vi" "Števec vseh skokov 4"(w521) -> ()
                  n217 = Add(x=w537, y=1.0) -> (x+y=w520:dbl)
                  n218 = Number To Decimal String(number=w519) -> (decimal integer string=w527:string)  [unwired: 1 in]
                  n219 = global write "Stevci_Globals.vi" "Števec skokov 4"(w520) -> ()
                  n220 = Concatenate Strings(w527, "igralec_skoki.tdms") -> (w525:string)
                  n221 = Replace Array Subset(array=w532, new element=w531, index (row)=w538) -> (w522:dbl[][])  [unwired: 1 in]
                  n222 = String To Path(string=w525) -> (path=w524:path)
                  n223 = Build Path(base path=w523, name or relative path=w524) -> (appended path=w530:path)
                  "appended path 4" <- w530
                  n224 = global write "Jumps_Globals.vi" "Jumps 4"(w522) -> ()
                  n225 = TDMS Open(10:T1."open or create" ("operation (0:open)"), 11:w530) -> (3:w535:refnum<k34>)  [unwired: 5 in, 1 out]
                  n226 = Decimal String To Number(string=w515) -> (number=w517:i32)  [unwired: 2 in, 1 out]
                  n227 = Decimal String To Number(string=w514) -> (number=w516:i32)  [unwired: 2 in, 1 out]
                  n228 = TDMS Write(0:w535, 5:"Skoki" ("group name in (Untitled)"), 7:w528, 9:w531) -> (4:w534:refnum<k34>)  [unwired: 2 in, 3 out]
                  n229 = Subtract(x=w517, y=w516) -> (x-y=w518:i32)
                  n230 = TDMS Close(11:w534) -> ()  [unwired: 1 in, 2 out]
                  n231 = global write "Stevci_Globals.vi" "casovna razlika"(w518) -> ()
                }
              }
            }
          }
          n232 = global write "belezenje.vi" "ID"(w448) -> ()
          "Sensor ID   4" <- w451
        }
        "Whole packet  4" <- w434
      }
      frame 5 {
        n233 = for {
          N: w543 -> [_]
          tunnel: w546 -> [w603]
          tunnel: w548 -> [w579]
          tunnel: w547 -> [w576]
          tunnel: w544 -> [w559]
          tunnel: w545 -> [w549]
          i -> [w562]
          w595 = 21
          n234 = global read "Stevci_Globals.vi" "Števec skokov 5"() -> (w554:dbl)
          n235 = Multiply(x=w595, y=w562) -> (x*y=w598:i32)
          n236 = Multiply(x=21, y=w562) -> (x*y=w600:i32)
          n237 = Multiply(x=w562, y=w595) -> (x*y=w602:i32)
          n238 = Add(x=37, y=w598) -> (x+y=w597:i32)
          n239 = Add(x=27, y=w602) -> (x+y=w593:i32)
          n240 = Add(x=22, y=w600) -> (x+y=w592:i32)
          n241 = String Subset(string=w603, offset (0)=w597, length (rest)=4) -> (substring=w591:string)
          "Flight time 5" <- w591
          n242 = String Subset(string=w579, offset (0)=12, length (rest)=8) -> (substring=w551:string)
          "Packet Time 5" <- w551
          n243 = String Subset(string=w576, offset (0)=2, length (rest)=4) -> (substring=w568:string)
          "Battery  5" <- w568
          n244 = String Subset(string=w603, offset (0)=w592, length (rest)=3) -> (substring=w560:string)
          "Jump ID 5" <- w560
          n245 = String Subset(string=w603, offset (0)=w593, length (rest)=8) -> (substring=w550:string)
          "Jump time  5" <- w550
          n246 = global read "Jump_Globals.vi" "Jump 5"() -> (w558:dbl[])
          n247 = Decimal String To Number(string=w551) -> (number=w583:i32)  [unwired: 2 in, 1 out]
          n248 = Decimal String To Number(string=w568) -> (number=w582:i32)  [unwired: 2 in, 1 out]
          n249 = Decimal String To Number(string=w591) -> (number=w589:i32)  [unwired: 2 in, 1 out]
          n250 = Decimal String To Number(string=w560) -> (number=w557:i32)  [unwired: 2 in, 1 out]
          n251 = Decimal String To Number(string=w550) -> (number=w590:i32)  [unwired: 2 in, 1 out]
          n252 = Replace Array Subset(array=w558, new element=w589, index=5) -> (w585:dbl[])
          n253 = Replace Array Subset(array=w585, new element=w590, index=4) -> (w575:dbl[])
          n254 = Replace Array Subset(array=w575, new element=w582, index=0) -> (w574:dbl[])
          n255 = Replace Array Subset(array=w574, new element=w583, index=1) -> (w573:dbl[])
          n256 = Replace Array Subset(array=w573, new element=w549, index=2) -> (w572:dbl[])
          n257 = Replace Array Subset(array=w572, new element=w557, index=3) -> (w555:dbl[])
          n258 = global write "Jump_Globals.vi" "Jump 5"(w555) -> ()
          n259 = global read "Jumps_Globals.vi" "Jumps 5"() -> (w553:dbl[][])
          n260 = Index Array(array=w553, index (col)=3 ("disabled index (col)")) -> (element=w566:dbl[])  [unwired: 1 in]
          n261 = Index Array(array=w553, index (row)=1) -> ()  [unwired: 1 in, 1 out]
          n262 = global write "belezenje.vi" "ID"(w549) -> ()
          n263 = Index Array(array=w555, index=3) -> (element=w564:dbl)
          n264 = for {
            tunnel: w566 -> [w649] mode=indexing
            tunnel: w564 -> [w648]
            tunnel: [w647] -> w563
            stop <- w647 stop-if-true
            n265 = Equal?(x=w649, y=w648) -> (x = y?=w647:bool)
          }
          n266 = Not(x=w563) -> (.not. x?=w561:bool)
          n267 = global read "filePath.vi" "Path"() -> (w552:path)
          n268 = case shown="True" w561 {
            tunnel: w553 -> [_ w618]
            tunnel: w555 -> [_ w617]
            tunnel: w554 -> [_ w620]
            tunnel: w554 -> [_ w619]
            tunnel: w560 -> [_ w616]
            tunnel: w549 -> [_ w615]
            tunnel: w552 -> [_ w614]
            tunnel: w557 -> [_ w611]
            tunnel: [0 w610] -> w556
            tunnel: w551 -> [_ w609]
            tunnel: w550 -> [_ w608]
            frame False {
            }
            frame True {
              n269 = global read "Stevci_Globals.vi" "Števec vseh skokov 5"() -> (w613:dbl)
              n270 = Greater?(x=w611, y=w613) -> (0:w612:bool)
              n271 = case shown="True" w612 {
                tunnel: w620 -> [_ w646]
                tunnel: w619 -> [_ w645]
                tunnel: w618 -> [_ w640]
                tunnel: w617 -> [_ w639]
                tunnel: w616 -> [_ w636]
                tunnel: w615 -> [_ w627]
                tunnel: w614 -> [_ w631]
                tunnel: w611 -> [_ w628]
                tunnel: [0 w627] -> w610
                tunnel: w609 -> [_ w623]
                tunnel: w608 -> [_ w622]
                frame False {
                }
                frame True {
                  n272 = Add(x=w645, y=1.0) -> (x+y=w629:dbl)
                  n273 = global write "Stevci_Globals.vi" "Števec vseh skokov 5"(w628) -> ()
                  n274 = global write "Stevci_Globals.vi" "Števec skokov 5"(w629) -> ()
                  n275 = Number To Decimal String(number=w627) -> (decimal integer string=w635:string)  [unwired: 1 in]
                  n276 = Concatenate Strings(w635, "igralec_skoki.tdms") -> (w633:string)
                  n277 = Replace Array Subset(array=w640, new element=w639, index (row)=w646) -> (w630:dbl[][])  [unwired: 1 in]
                  n278 = global write "Jumps_Globals.vi" "Jumps 5"(w630) -> ()
                  n279 = String To Path(string=w633) -> (path=w632:path)
                  n280 = Build Path(base path=w631, name or relative path=w632) -> (appended path=w638:path)
                  "appended path 5" <- w638
                  n281 = TDMS Open(10:T1."open or create" ("operation (0:open)"), 11:w638) -> (3:w643:refnum<k34>)  [unwired: 5 in, 1 out]
                  n282 = TDMS Write(0:w643, 5:"Skoki" ("group name in (Untitled)"), 7:w636, 9:w639) -> (4:w642:refnum<k34>)  [unwired: 2 in, 3 out]
                  n283 = Decimal String To Number(string=w623) -> (number=w625:i32)  [unwired: 2 in, 1 out]
                  n284 = Decimal String To Number(string=w622) -> (number=w624:i32)  [unwired: 2 in, 1 out]
                  n285 = TDMS Close(11:w642) -> ()  [unwired: 1 in, 2 out]
                  n286 = Subtract(x=w625, y=w624) -> (x-y=w626:i32)
                  n287 = global write "Stevci_Globals.vi" "casovna razlika"(w626) -> ()
                }
              }
            }
          }
          n288 = global write "belezenje.vi" "ID"(w556) -> ()
          "Sensor ID   5" <- w559
        }
        "Whole packet 5  2" <- w542
      }
      frame 6 {
        n289 = for {
          N: w651 -> [_]
          tunnel: w653 -> [w711]
          tunnel: w656 -> [w687]
          tunnel: w654 -> [w684]
          tunnel: w652 -> [w667]
          tunnel: w655 -> [w657]
          i -> [w670]
          w703 = 21
          n290 = global read "Stevci_Globals.vi" "Števec skokov 6"() -> (w661:dbl)
          n291 = Multiply(x=w703, y=w670) -> (x*y=w706:i32)
          n292 = Multiply(x=21, y=w670) -> (x*y=w708:i32)
          n293 = Multiply(x=w670, y=w703) -> (x*y=w710:i32)
          n294 = Add(x=37, y=w706) -> (x+y=w705:i32)
          n295 = Add(x=27, y=w710) -> (x+y=w701:i32)
          n296 = Add(x=22, y=w708) -> (x+y=w700:i32)
          n297 = String Subset(string=w711, offset (0)=w705, length (rest)=4) -> (substring=w699:string)
          "Flight time 6" <- w699
          n298 = String Subset(string=w687, offset (0)=12, length (rest)=8) -> (substring=w659:string)
          "Packet Time 6" <- w659
          n299 = String Subset(string=w684, offset (0)=2, length (rest)=4) -> (substring=w676:string)
          "Battery  6" <- w676
          n300 = String Subset(string=w711, offset (0)=w700, length (rest)=3) -> (substring=w668:string)
          "Jump ID 6" <- w668
          n301 = String Subset(string=w711, offset (0)=w701, length (rest)=8) -> (substring=w658:string)
          "Jump time  6" <- w658
          n302 = Decimal String To Number(string=w659) -> (number=w691:i32)  [unwired: 2 in, 1 out]
          n303 = Decimal String To Number(string=w676) -> (number=w690:i32)  [unwired: 2 in, 1 out]
          n304 = Decimal String To Number(string=w699) -> (number=w697:i32)  [unwired: 2 in, 1 out]
          n305 = Decimal String To Number(string=w668) -> (number=w665:i32)  [unwired: 2 in, 1 out]
          n306 = Decimal String To Number(string=w658) -> (number=w698:i32)  [unwired: 2 in, 1 out]
          n307 = global read "Jump_Globals.vi" "Jump 6"() -> (w666:dbl[])
          n308 = Replace Array Subset(array=w666, new element=w697, index=5) -> (w693:dbl[])
          n309 = Replace Array Subset(array=w693, new element=w698, index=4) -> (w683:dbl[])
          n310 = Replace Array Subset(array=w683, new element=w690, index=0) -> (w682:dbl[])
          n311 = Replace Array Subset(array=w682, new element=w691, index=1) -> (w681:dbl[])
          n312 = Replace Array Subset(array=w681, new element=w657, index=2) -> (w680:dbl[])
          n313 = Replace Array Subset(array=w680, new element=w665, index=3) -> (w663:dbl[])
          n314 = global write "Jump_Globals.vi" "Jump 6"(w663) -> ()
          n315 = global read "Jumps_Globals.vi" "Jumps 6"() -> (w662:dbl[][])
          n316 = Index Array(array=w662, index (col)=3 ("disabled index (col)")) -> (element=w674:dbl[])  [unwired: 1 in]
          n317 = Index Array(array=w662, index (row)=1) -> ()  [unwired: 1 in, 1 out]
          n318 = global write "belezenje.vi" "ID"(w657) -> ()
          n319 = Index Array(array=w663, index=3) -> (element=w672:dbl)
          n320 = for {
            tunnel: w674 -> [w757] mode=indexing
            tunnel: w672 -> [w756]
            tunnel: [w755] -> w671
            stop <- w755 stop-if-true
            n321 = Equal?(x=w757, y=w756) -> (x = y?=w755:bool)
          }
          n322 = Not(x=w671) -> (.not. x?=w669:bool)
          n323 = global read "filePath.vi" "Path"() -> (w660:path)
          n324 = case shown="True" w669 {
            tunnel: w662 -> [_ w726]
            tunnel: w663 -> [_ w725]
            tunnel: w661 -> [_ w728]
            tunnel: w661 -> [_ w727]
            tunnel: w668 -> [_ w724]
            tunnel: w657 -> [_ w723]
            tunnel: w660 -> [_ w722]
            tunnel: w665 -> [_ w719]
            tunnel: [0 w718] -> w664
            tunnel: w659 -> [_ w717]
            tunnel: w658 -> [_ w716]
            frame False {
            }
            frame True {
              n325 = global read "Stevci_Globals.vi" "Števec vseh skokov 6"() -> (w721:dbl)
              n326 = Greater?(x=w719, y=w721) -> (0:w720:bool)
              n327 = case shown="True" w720 {
                tunnel: w728 -> [_ w754]
                tunnel: w727 -> [_ w753]
                tunnel: w726 -> [_ w748]
                tunnel: w725 -> [_ w747]
                tunnel: w724 -> [_ w744]
                tunnel: w723 -> [_ w735]
                tunnel: w722 -> [_ w739]
                tunnel: w719 -> [_ w737]
                tunnel: [0 w735] -> w718
                tunnel: w717 -> [_ w732]
                tunnel: w716 -> [_ w733]
                frame False {
                }
                frame True {
                  n328 = global write "Stevci_Globals.vi" "Števec vseh skokov 6"(w737) -> ()
                  n329 = Add(x=w753, y=1.0) -> (x+y=w736:dbl)
                  n330 = global write "Stevci_Globals.vi" "Števec skokov 6"(w736) -> ()
                  n331 = Number To Decimal String(number=w735) -> (decimal integer string=w743:string)  [unwired: 1 in]
                  n332 = Replace Array Subset(array=w748, new element=w747, index (row)=w754) -> (w738:dbl[][])  [unwired: 1 in]
                  n333 = Concatenate Strings(w743, "igralec_skoki.tdms") -> (w741:string)
                  n334 = global write "Jumps_Globals.vi" "Jumps 6"(w738) -> ()
                  n335 = String To Path(string=w741) -> (path=w740:path)
                  n336 = Build Path(base path=w739, name or relative path=w740) -> (appended path=w746:path)
                  "appended path 6" <- w746
                  n337 = TDMS Open(10:T1."open or create" ("operation (0:open)"), 11:w746) -> (3:w751:refnum<k34>)  [unwired: 5 in, 1 out]
                  n338 = TDMS Write(0:w751, 5:"Skoki" ("group name in (Untitled)"), 7:w744, 9:w747) -> (4:w750:refnum<k34>)  [unwired: 2 in, 3 out]
                  n339 = TDMS Close(11:w750) -> ()  [unwired: 1 in, 2 out]
                  n340 = Decimal String To Number(string=w732) -> (number=w731:i32)  [unwired: 2 in, 1 out]
                  n341 = Decimal String To Number(string=w733) -> (number=w730:i32)  [unwired: 2 in, 1 out]
                  n342 = Subtract(x=w731, y=w730) -> (x-y=w734:i32)
                  n343 = global write "Stevci_Globals.vi" "casovna razlika"(w734) -> ()
                }
              }
            }
          }
          n344 = global write "belezenje.vi" "ID"(w664) -> ()
          "Sensor ID   6" <- w667
        }
        "Whole packet 6  2" <- w650
      }
    }
    n345 = String Subset(string=w10, offset (0)=2, length (rest)=4) -> (substring=w14:string)
    n346 = case shown="1" w17 {
      tunnel: w14 -> [_ w32 w46 w60 w74 w87 w100]
      frame 0, Default {
      }
      frame 1 {
        n347 = Tick Count (ms)() -> (millisecond timer value=w33:u32)
        n348 = Decimal String To Number(string=w32) -> (number=w30:i32)  [unwired: 2 in, 1 out]
        n349 = To Double Precision Float(number=w30) -> (double precision float=w29:dbl)
        n350 = global write "senzorji.vi" "1"(TRUE ("1")) -> ()
        n351 = global write "senzorji.vi" "Numeric"(w33) -> ()
        n352 = xnode "Formula"("X1"=w29) -> ("Result"=w31:dbl)  [unwired: 1 in, 1 out]
        n353 = global write "senzorji.vi" "bat 1"(w31) -> ()
      }
      frame 2 {
        n354 = Decimal String To Number(string=w46) -> (number=w44:i32)  [unwired: 2 in, 1 out]
        n355 = Tick Count (ms)() -> (millisecond timer value=w47:u32)
        n356 = global write "senzorji.vi" "2"(TRUE ("2")) -> ()
        n357 = To Double Precision Float(number=w44) -> (double precision float=w43:dbl)
        n358 = global write "senzorji.vi" "Numeric 2"(w47) -> ()
        n359 = xnode "Formula"("X1"=w43) -> ("Result"=w45:dbl)  [unwired: 1 in, 1 out]
        n360 = global write "senzorji.vi" "bat 2"(w45) -> ()
      }
      frame 3 {
        n361 = Decimal String To Number(string=w60) -> (number=w58:i32)  [unwired: 2 in, 1 out]
        n362 = Tick Count (ms)() -> (millisecond timer value=w61:u32)
        n363 = To Double Precision Float(number=w58) -> (double precision float=w57:dbl)
        n364 = global write "senzorji.vi" "3"(TRUE ("3")) -> ()
        n365 = global write "senzorji.vi" "Numeric 3"(w61) -> ()
        n366 = xnode "Formula"("X1"=w57) -> ("Result"=w59:dbl)  [unwired: 1 in, 1 out]
        n367 = global write "senzorji.vi" "bat 3"(w59) -> ()
      }
      frame 4 {
        n368 = Decimal String To Number(string=w74) -> (number=w72:i32)  [unwired: 2 in, 1 out]
        n369 = Tick Count (ms)() -> (millisecond timer value=w75:u32)
        n370 = To Double Precision Float(number=w72) -> (double precision float=w71:dbl)
        n371 = global write "senzorji.vi" "4"(TRUE ("3")) -> ()
        n372 = xnode "Formula"("X1"=w71) -> ("Result"=w73:dbl)  [unwired: 1 in, 1 out]
        n373 = global write "senzorji.vi" "Numeric 4"(w75) -> ()
        n374 = global write "senzorji.vi" "bat 4"(w73) -> ()
      }
      frame 5 {
        n375 = Decimal String To Number(string=w87) -> (number=w86:i32)  [unwired: 2 in, 1 out]
        n376 = Tick Count (ms)() -> (millisecond timer value=w88:u32)
        n377 = global write "senzorji.vi" "5"(TRUE ("3")) -> ()
        n378 = global write "senzorji.vi" "Numeric 5"(w88) -> ()
        n379 = xnode "Formula"("X1"=w86) -> ("Result"=w85:dbl)  [unwired: 1 in, 1 out]
        n380 = global write "senzorji.vi" "bat 5"(w85) -> ()
      }
      frame 6 {
        n381 = Tick Count (ms)() -> (millisecond timer value=w101:u32)
        n382 = Decimal String To Number(string=w100) -> (number=w99:i32)  [unwired: 2 in, 1 out]
        n383 = xnode "Formula"("X1"=w99) -> ("Result"=w98:dbl)  [unwired: 1 in, 1 out]
        n384 = global write "senzorji.vi" "Numeric 6"(w101) -> ()
        n385 = global write "senzorji.vi" "6"(TRUE ("3")) -> ()
        n386 = global write "senzorji.vi" "bat 6"(w98) -> ()
      }
    }
  }
  n387 = Initialize Array(0.0 ("element"), 6 ("dimension size")) -> (w1:dbl[])
  n388 = global write "Jump_Globals.vi" "Jump 5"(w1) -> ()
  n389 = global write "Jump_Globals.vi" "Jump 6"(w1) -> ()
  n390 = global write "Jump_Globals.vi" "Jump 2"(w1) -> ()
  n391 = global write "Jump_Globals.vi" "Jump 3"(w1) -> ()
  n392 = global write "Jump_Globals.vi" "Jump 4"(w1) -> ()
  n393 = global write "Jump_Globals.vi" "Jump 1"(w1) -> ()
  n394 = UDP Close(connection ID=w7, 8:w5) -> (error out=w6:errorcluster)  [unwired: 1 out]
  n395 = call <vilib>:"Simple Error Handler.vi"("error in (no error)"=w6) -> ()  [unwired: 1 in, 8 out]
